vi "Tektronix TDS 3000 Series Wait For Acquisition Complete Example.vi"() -> ()   [LabVIEW 2010]
doc: "DESCRIPTION:\nThis example shows how to properly use the Wait For Acquisition Complete VI to acquire large waveforms from the Tektronix TDS 3xxx Series scopes.\n\nINSTRUCTIONS:\n1. Pass a valid VISA session.\n2. Enter the desired channel.\n3. The acquired waveform will be displayed in the graph."
uses:
  <instrlib>/Tektronix TDS 3000 Series/Tektronix TDS 3000 Series.lvlib
panel:
  in  "Maximum Time (10000 ms)":u32=10000
  out "Waveform Graph":T1(graph)
  in  "VISA Resource Name":refnum<visa-resource-name>="GPIB0::1::INSTR"
  in  "Channel (\"CH1\")":string(combo)="CH1"
  # "© 2003-2007, National Instruments, Corporation.  All Rights Reserved."
  # "For instructions,\nselect Show Context Help\nfrom the Help menu."
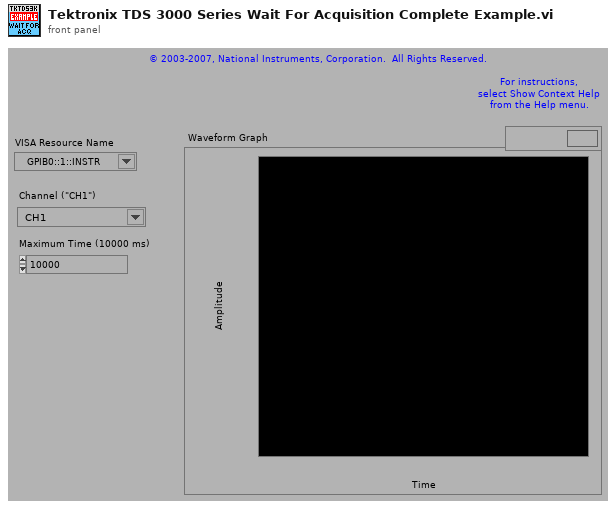
[diagram p1: front panel]
types:
  T1 = cluster{"Initial X":dbl, "X Increment":dbl, "Waveform Array":dbl[]}
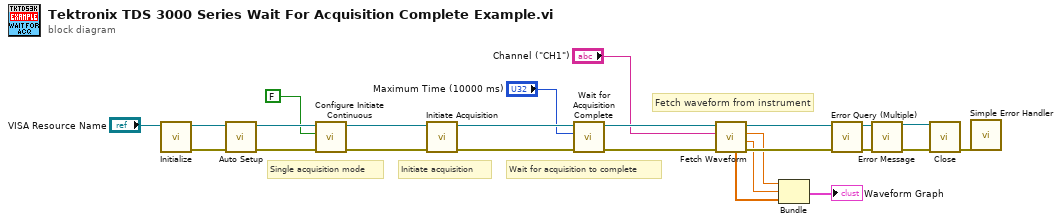
[diagram p0: block diagram]
diagram:
  # "Fetch waveform from instrument"
  # "Wait for acquisition to complete"
  # "Initiate acquisition"
  # "Single acquisition mode"
  n1 = call <instrlib>:"Initialize.vi"("VISA Resource Name"="VISA Resource Name") -> ("error out"=w25:errorcluster, "VISA Resource Name Out"=w24:refnum<visa-resource-name>)  [unwired: 9 in]
  n2 = call <instrlib>:"Auto Setup.vi"("error in (no error)"=w25, "VISA Resource Name"=w24) -> ("error out"=w23:errorcluster, "VISA Resource Name Out"=w22:refnum<visa-resource-name>)  [unwired: 8 in]
  n3 = call <instrlib>:"Configure Initiate Continuous.vi"("error in (no error)"=w23, "Continuous Acquisition (False)"=FALSE, "VISA Resource Name"=w22) -> ("error out"=w20:errorcluster, "VISA Resource Name Out"=w19:refnum<visa-resource-name>)  [unwired: 7 in]
  n4 = call <instrlib>:"Initiate Acquisition.vi"("error in (no error)"=w20, "VISA Resource Name"=w19) -> ("error out"=w18:errorcluster, "VISA Resource Name Out"=w17:refnum<visa-resource-name>)  [unwired: 8 in]
  n5 = call <instrlib>:"Wait for Acquisition Complete.vi"("error in (no error)"=w18, "Maximum Time (10000 ms)"="Maximum Time (10000 ms)", "VISA Resource Name"=w17) -> ("error out"=w16:errorcluster, "VISA Resource Name Out"=w15:refnum<visa-resource-name>)  [unwired: 7 in]
  n6 = call <instrlib>:"Fetch Waveform.vi"("error in (no error)"=w16, "Source (Channel 1)"="Channel (\"CH1\")", "VISA Resource Name"=w15) -> ("error out"=w13:errorcluster, "X Increment"=w5:dbl, "Initial X"=w6:dbl, "VISA Resource Name Out"=w12:refnum<visa-resource-name>, "Waveform Array"=w4:dbl[])  [unwired: 3 in, 1 out]
  n7 = Bundle("Initial X"=w6, "X Increment"=w5, "Waveform Array"=w4) -> (→"Waveform Graph":T1)  [unwired: 1 in]
  n8 = call <instrlib>:"Error Query (Multiple).vi"("error in (no error)"=w13, "VISA Resource Name"=w12) -> ("error out"=w10:errorcluster, "VISA Resource Name Out"=w11:refnum<visa-resource-name>)  [unwired: 6 in, 2 out]
  n9 = call <instrlib>:"Error Message.vi"("VISA Resource Name"=w11, "error in (no error)"=w10) -> ("VISA Resource Name Out"=w8:refnum<visa-resource-name>, "error out"=w9:errorcluster)  [unwired: 9 in, 3 out]
  n10 = call <instrlib>:"Close.vi"("error in (no error)"=w9, "VISA Resource Name"=w8) -> ("error out"=w1:errorcluster)  [unwired: 9 in]
  n11 = call <vilib>:"Simple Error Handler.vi"("error in (no error)"=w1) -> ()  [unwired: 4 in, 5 out]
